vi "Read Type.vi"(8 "error in (no error)":errorcluster, 11 "_Shared in":refnum<class "_Shared.lvclass">) -> (0 "error out":errorcluster, 2 "Type":string, 3 "_Shared out":refnum<class "_Shared.lvclass">)   [LabVIEW 2021, in "_Rename.lvlib" / "_Shared.lvclass"]
uses:
  _Shared.lvclass
  _Shared.lvclass/_Shared.ctl
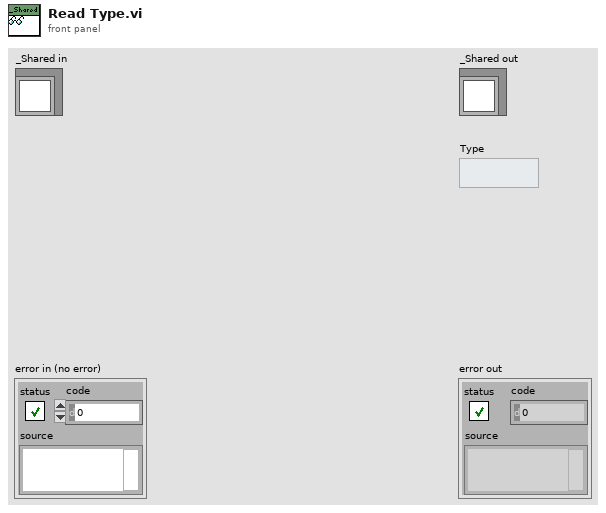
[diagram p1: front panel]
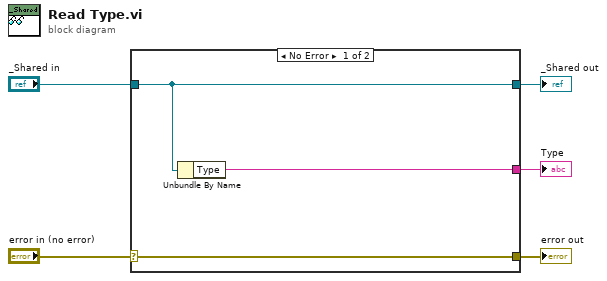
[diagram p0: block diagram]
diagram:
  n1 = case shown="No Error" "error in (no error)" {
    selector: "error in (no error)" -> [w8 w9]
    tunnel: [w8 w9] -> w4
    tunnel: [w7 w10] -> w2
    tunnel: "_Shared in" -> [w7 w10]
    tunnel: [w6 _] -> w1
    frame No Error {
      n2 = Unbundle By Name(w7) -> ("Type"=w6:string)
    }
    frame Error {
    }
  }
  "error out" <- w4
  "_Shared out" <- w2
  "Type" <- w1
